vi "accounts_file_access.vi"(6 "AccountCommand":T1, 7 "error in (no error)":errorcluster, 9 "Amount":dbl, 10 "Account":string) -> (0 "error out":errorcluster, 2 "Value Out":string)   [LabVIEW 2017]
uses:
  controls/AccountCmd.ctl
  <vilib>/Utility/file.llb/Read From Spreadsheet File (string).vi
  <vilib>/Utility/file.llb/Write To Spreadsheet File (string).vi
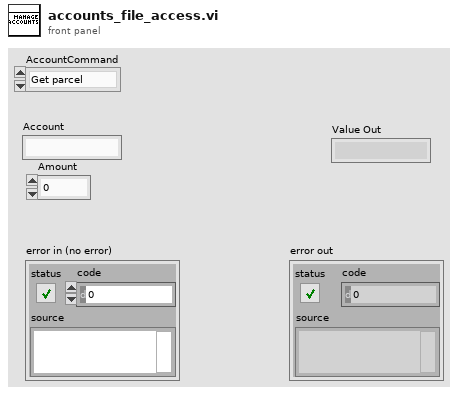
[diagram p1: front panel]
types:
  T1 = typedef "AccountCmd.ctl" = enum16{"Get parcel", "Get number", "Deposit", "Withdrawal"}
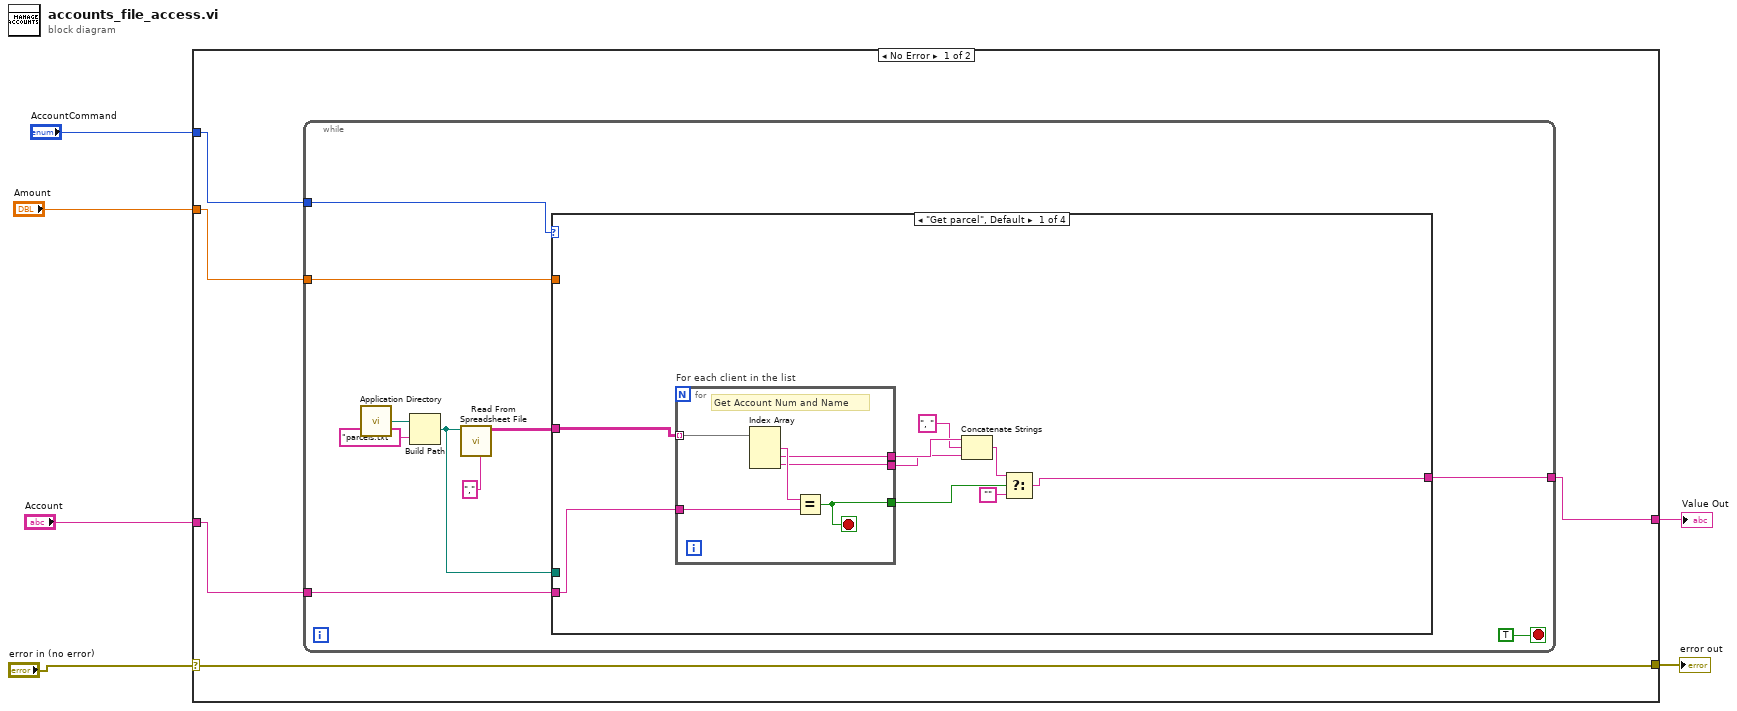
[diagram p0: block diagram]
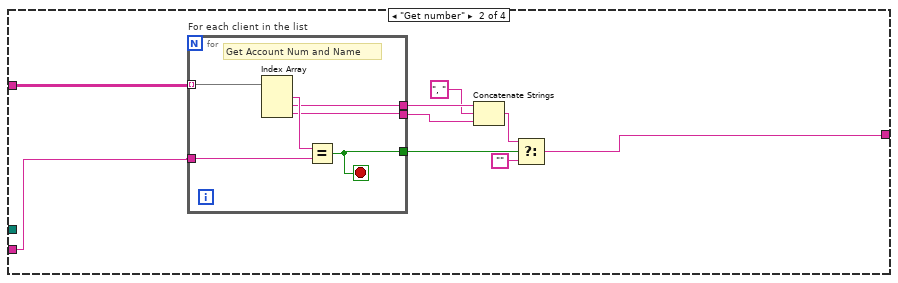
[diagram p2: hidden frame]
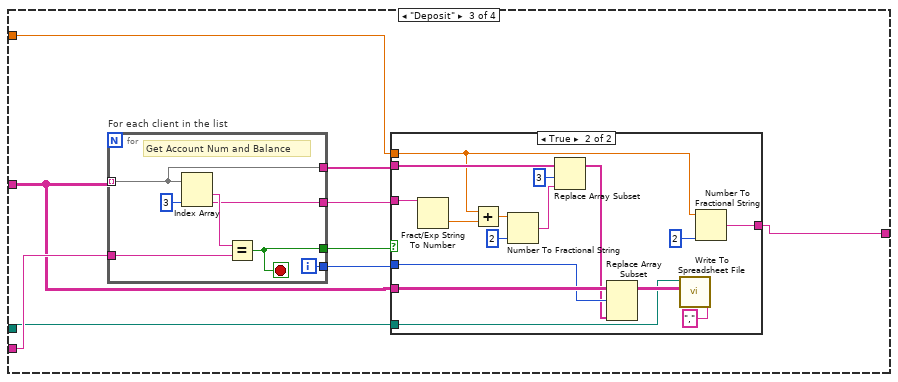
[diagram p3: hidden frame]
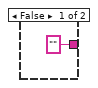
[diagram p4: hidden frame]
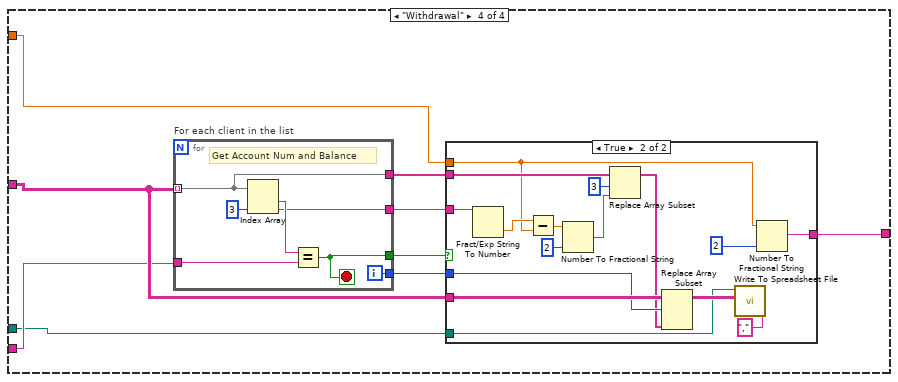
[diagram p5: hidden frame]
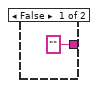
[diagram p6: hidden frame]
diagram:
  n1 = case shown="No Error" "error in (no error)" {
    selector: "error in (no error)" -> [w8 w118]
    tunnel: [w7 w119] -> w4
    tunnel: "Account" -> [w9 w119]
    tunnel: [w8 w118] -> w3
    tunnel: "Amount" -> [w10 _]
    tunnel: "AccountCommand" -> [w11 _]
    frame No Error {
      n2 = while {
        tunnel: w9 -> [w18]
        tunnel: w11 -> [w17]
        tunnel: w10 -> [w16]
        tunnel: [w13] -> w7
        stop <- TRUE stop-if-true
        n3 = call <vilib>:"Application Directory.vi"() -> ("Application Directory"=w21:path)
        n4 = Build Path(base path=w21, name or relative path="parcels.txt") -> (appended path=w15:path)
        n5 = call-poly <vilib>:"Read From Spreadsheet File.vi"("delimiter (\\t)"="," ("delimiter (\\t)"), "file path (dialog if empty)"=w15) -> ("all rows"=w14:string[][])  [unwired: 5 in, 4 out]
        n6 = case shown="\"Get parcel\", Default" w17 {
          tunnel: w18 -> [w24 w38 w60 w86]
          tunnel: w16 -> [_ _ w57 w88]
          tunnel: w15 -> [_ _ w55 w85]
          tunnel: w14 -> [w23 w37 w53 w87]
          tunnel: [w22 w39 w56 w89] -> w13
          frame "Get parcel", Default {
            n7 = for "For each client in the list" {
              tunnel: w24 -> [w36]
              tunnel: [w35] -> w30
              tunnel: [w32] -> w27
              tunnel: [w31] -> w26
              tunnel: w23 -> [w34] mode=indexing
              stop <- w35 stop-if-true
              # "Get Account Num and Name"
              n8 = Index Array(array=w34) -> (element #1=w33:string, element #2=w32:string, element #3=w31:string)  [unwired: 3 in]
              n9 = Equal?(x=w33, y=w36) -> (x = y?=w35:bool)
            }
            n10 = Concatenate Strings(w27, ", " ("string"), w26) -> (w28:string)
            n11 = Select(t=w28, s=w30, f="") -> (s? t:f=w22:string)
          }
          frame "Get number" {
            n12 = for "For each client in the list" {
              tunnel: w38 -> [w51]
              tunnel: [w50] -> w45
              tunnel: [w47] -> w42
              tunnel: [w46] -> w41
              tunnel: w37 -> [w49] mode=indexing
              stop <- w50 stop-if-true
              # "Get Account Num and Name"
              n13 = Index Array(array=w49) -> (element #1=w48:string, element #2=w47:string, element #3=w46:string)  [unwired: 3 in]
              n14 = Equal?(x=w48, y=w51) -> (x = y?=w50:bool)
            }
            n15 = Concatenate Strings(w42, ", " ("string"), w41) -> (w43:string)
            n16 = Select(t=w43, s=w45, f="") -> (s? t:f=w39:string)
          }
          frame "Deposit" {
            n17 = for "For each client in the list" {
              tunnel: w60 -> [w84]
              tunnel: [w83] -> w52
              tunnel: w53 -> [w79] mode=indexing
              tunnel: [w80] -> w59
              tunnel: [w79] -> w58
              tunnel: [w78] -> w54
              i -> [w78]
              stop <- w83 stop-if-true
              # "Get Account Num and Balance"
              n18 = Index Array(array=w79, index #2=3 ("index")) -> (element #1=w82:string, element #2=w80:string)  [unwired: 1 in]
              n19 = Equal?(x=w82, y=w84) -> (x = y?=w83:bool)
            }
            n20 = case shown="True" w52 {
              tunnel: w59 -> [_ w66]
              tunnel: w57 -> [_ w64]
              tunnel: w58 -> [_ w75]
              tunnel: w53 -> [_ w73]
              tunnel: w54 -> [_ w72]
              tunnel: w55 -> [_ w69]
              tunnel: ["" w65] -> w56
              frame False {
              }
              frame True {
                n21 = Fract/Exp String To Number(string=w66) -> (number=w77:dbl)  [unwired: 3 in, 1 out]
                n22 = Add(x=w64, y=w77) -> (x+y=w76:dbl)
                n23 = Number To Fractional String(number=w76, precision (6)=i16 2) -> (F-format string=w67:string)  [unwired: 2 in]
                n24 = Replace Array Subset(array=w75, new element=w67, index=3) -> (w71:string[])
                n25 = Replace Array Subset(array=w73, new element=w71, index (row)=w72) -> (w70:string[][])  [unwired: 1 in]
                n26 = call-poly <vilib>:"Write To Spreadsheet File.vi"("delimiter (\\t)"="," ("delimiter (\\t)"), "2D data"=w70, "file path (dialog if empty)"=w69) -> ()  [unwired: 5 in, 1 out]
                n27 = Number To Fractional String(number=w64, precision (6)=i16 2) -> (F-format string=w65:string)  [unwired: 2 in]
              }
            }
          }
          frame "Withdrawal" {
            n28 = for "For each client in the list" {
              tunnel: w86 -> [w117]
              tunnel: [w116] -> w92
              tunnel: w87 -> [w112] mode=indexing
              tunnel: [w113] -> w93
              tunnel: [w112] -> w91
              tunnel: [w111] -> w90
              i -> [w111]
              stop <- w116 stop-if-true
              # "Get Account Num and Balance"
              n29 = Index Array(array=w112, index #2=3 ("index")) -> (element #1=w115:string, element #2=w113:string)  [unwired: 1 in]
              n30 = Equal?(x=w115, y=w117) -> (x = y?=w116:bool)
            }
            n31 = case shown="True" w92 {
              tunnel: w93 -> [_ w99]
              tunnel: w88 -> [_ w97]
              tunnel: w91 -> [_ w110]
              tunnel: w87 -> [_ w108]
              tunnel: w90 -> [_ w107]
              tunnel: w85 -> [_ w104]
              tunnel: ["" w98] -> w89
              frame False {
              }
              frame True {
                n32 = Fract/Exp String To Number(string=w99) -> (number=w101:dbl)  [unwired: 3 in, 1 out]
                n33 = Subtract(x=w101, y=w97) -> (x-y=w100:dbl)
                n34 = Number To Fractional String(number=w100, precision (6)=i16 2) -> (F-format string=w102:string)  [unwired: 2 in]
                n35 = Replace Array Subset(array=w110, new element=w102, index=3) -> (w106:string[])
                n36 = Replace Array Subset(array=w108, new element=w106, index (row)=w107) -> (w105:string[][])  [unwired: 1 in]
                n37 = call-poly <vilib>:"Write To Spreadsheet File.vi"("delimiter (\\t)"="," ("delimiter (\\t)"), "2D data"=w105, "file path (dialog if empty)"=w104) -> ()  [unwired: 5 in, 1 out]
                n38 = Number To Fractional String(number=w97, precision (6)=i16 2) -> (F-format string=w98:string)  [unwired: 2 in]
              }
            }
          }
        }
      }
    }
    frame Error {
    }
  }
  "error out" <- w3
  "Value Out" <- w4
